vi "DbFetchRecoedSetFromFile.vi"() -> ()   [LabVIEW 2019]
uses:
  <vilib>/addons/database/Connection.llb/DB Tools Open Connec (String).vi
  <vilib>/addons/database/Recordset.llb/Rec Fetch Recordset Data (R).vi
  <vilib>/addons/database/NI_Database_API.lvlib
panel:
  in  "Write Your ODBC Server Name here":string
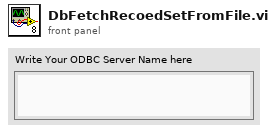
[diagram p1: front panel]
types:
  T1 = typedef "NI_Database_API.lvlib/Conn ObjectReference.ctl" = refnum<k1>
  T2 = typedef "NI_Database_API.lvlib/Rec ObjectReference.ctl" = refnum<k1>
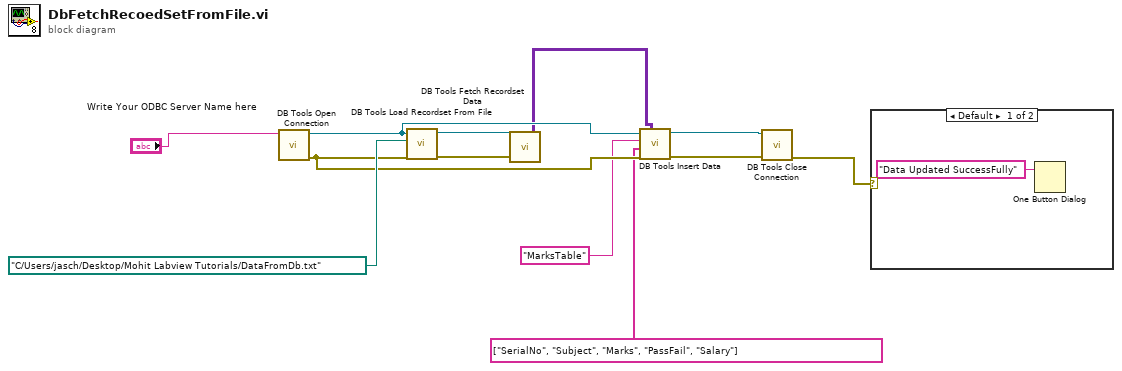
[diagram p0: block diagram]
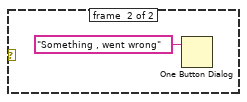
[diagram p2: hidden frame]
diagram:
  n1 = call-poly <vilib>:"DB Tools Open Connection.vi"("connection information"="Write Your ODBC Server Name here") -> ("error out"=w6:errorcluster, "connection reference"=w8:T1)  [unwired: 7 in]
  n2 = call <vilib>:"DB Tools Load Recordset From File.vi"("error in (no error)"=w6, "file name"=path "C:/Users/jasch/Desktop/Mohit Labview Tutorials/DataFromDb.txt", "connection reference"=w8) -> ("error out"=w10:errorcluster, "recordset reference"=w9:T2)  [unwired: 3 in]
  n3 = call-poly <vilib>:"DB Tools Fetch Recordset Data.vi"("error in (no error)"=w10, "recordset reference"=w9) -> ("recordset data"=w7:variant[][])  [unwired: 3 in, 2 out]
  n4 = call <vilib>:"DB Tools Insert Data.vi"("data"=w7, "error in (no error)"=w6, "columns"=string[] ["SerialNo", "Subject", "Marks", "PassFail", "Salary"], "table"="MarksTable", "connection reference"=w8) -> ("error out"=w2:errorcluster, "connection reference out"=w3:T1)  [unwired: 5 in]
  n5 = call <vilib>:"DB Tools Close Connection.vi"("error in (no error)"=w2, "connection reference"=w3) -> ("error out"=w1:errorcluster)  [unwired: 5 in]
  n6 = case shown="Default" w1 {
    frame #0 {
      n7 = One Button Dialog(message="Data Updated SuccessFully") -> ()  [unwired: 1 in, 1 out]
    }
    frame #1 {
      n8 = One Button Dialog(message="Something , went wrong") -> ()  [unwired: 1 in, 1 out]
    }
  }
